vi "Resolve Path.vi"(10 "Path":string, 11 "Base Dir":path) -> (3 "Resolved Path":path)   [LabVIEW 2022 SP3, in "Core.lvlib" / "Config.lvlib"]
uses:
  Config.lvlib
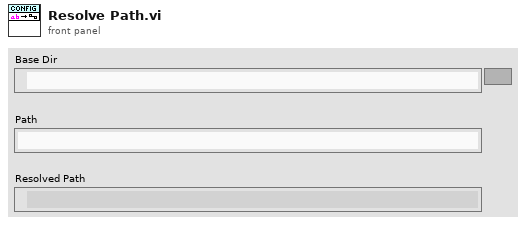
[diagram p1: front panel]
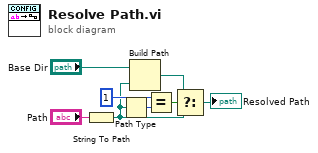
[diagram p0: block diagram]
diagram:
  n1 = String To Path(string="Path") -> (path=w4:path)
  n2 = Path Type(1:w4) -> (0:w8:i16)
  n3 = Build Path(base path="Base Dir", name or relative path=w4) -> (appended path=w5:path)
  n4 = Equal?(x=i16 1 ("y"), y=w8) -> (x = y?=w6:bool)
  n5 = Select(t=w5, s=w6, f=w4) -> (s? t:f=→"Resolved Path":path)
